vi "Test Add Event Registration.vi"   [LabVIEW 2020, in "TEST JKI State Machine API.lvlib"]
uses:
  TEST JKI State Machine API.lvlib
  source/JKI SM/JKI SM.lvclass
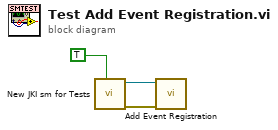
[diagram p0: block diagram]
diagram:
  n1 = call "New JKI sm for Tests.vi"("Open SM FP (for debugging)"=TRUE) -> ("error out"=w1:errorcluster, "JKI SM out"=w2:refnum<class "JKI SM.lvclass">)  [unwired: 9 in]
  n2 = call-dynamic "Add Event Registration.vi"("error in (no error)"=w1, "JKI SM in"=w2) -> ()  [unwired: 8 in, 2 out]
